vi "Initialize.vi"(8 "error in (no error)":errorcluster, 11 "View Template in":refnum<class "Logger Normal.lvclass">) -> (0 "error out":errorcluster, 3 "View Template out":refnum<class "Logger Normal.lvclass">)   [LabVIEW 2020, in "Logger Normal.lvlib" / "Logger Normal.lvclass"]
uses:
  Logger Normal.lvclass
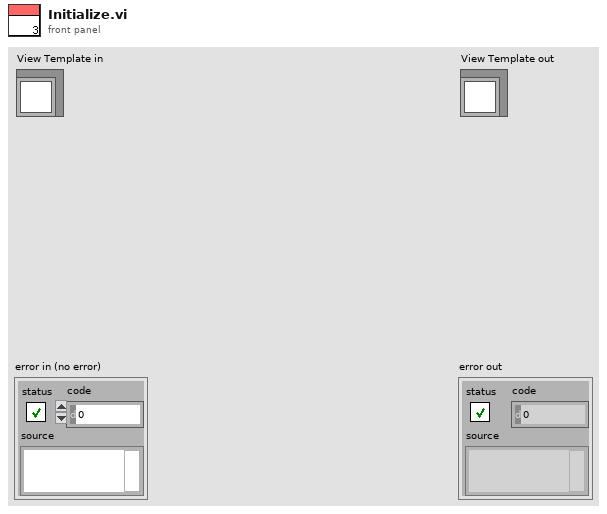
[diagram p1: front panel]
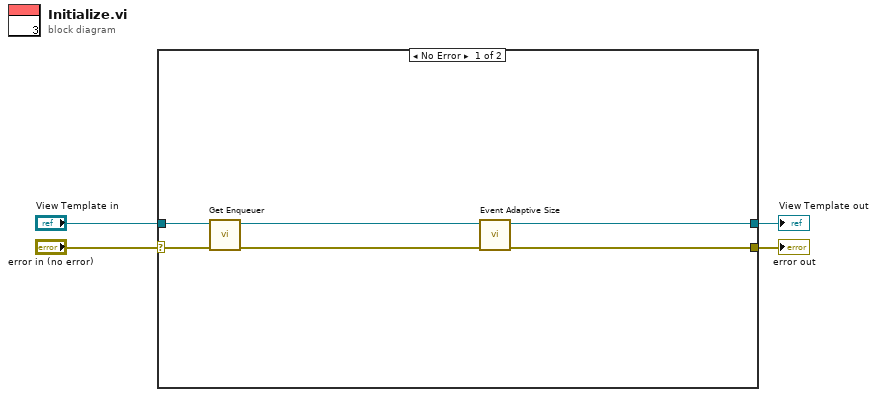
[diagram p0: block diagram]
diagram:
  n1 = case shown="No Error" "error in (no error)" {
    selector: "error in (no error)" -> [w9 w12]
    tunnel: [w7 w12] -> w3
    tunnel: [w5 w11] -> w1
    tunnel: "View Template in" -> [w10 w11]
    frame No Error {
      n2 = call "Get Enqueuer.vi"("error in (no error)"=w9, "View Template in"=w10) -> ("error out"=w8:errorcluster, "View Template out"=w6:refnum<class "Logger Normal.lvclass">)  [unwired: 8 in]
      n3 = call "Event Adaptive Size.vi"("error in (no error)"=w8, "Logger Normal in"=w6) -> ("error out"=w7:errorcluster, "Logger Normal out"=w5:refnum<class "Logger Normal.lvclass">)  [unwired: 8 in]
    }
    frame Error {
    }
  }
  "error out" <- w3
  "View Template out" <- w1
